vi "Reset Encoder_1.vi"(2 "DC Motors":cluster{"DC Motor":T1, "Address":i16}={"DC Motor"=enum."DC Motor", "Address"=-1}, 3 "NXT":T2={"Hardware"="NXT", "Flattened String"=""}) -> (0 "NXT":T2={"Hardware"="NXT", "Flattened String"=""})   [LabVIEW 2010, in "4134Outputs.lvlib"]
uses:
  4134Outputs.lvlib
  <vilib>/NXT/Subs/LVHSConnector.ctl
  <vilib>/NXT/Subs/MotorXNode.DC Motor Type.ctl
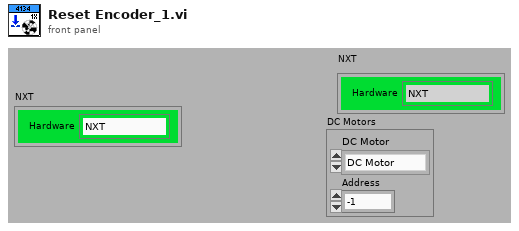
[diagram p1: front panel]
types:
  T1 = typedef "MotorXNode.DC Motor Type.ctl" = enum16{"DC Motor"}
  T2 = typedef "LVHSConnector.ctl" = cluster{"Hardware":string, "Flattened String":string}
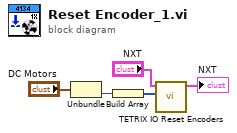
[diagram p0: block diagram]
diagram:
  n1 = Unbundle("DC Motors") -> ("Address"=w5:i16)  [unwired: 1 out]
  n2 = Build Array(w5) -> (w2:i16[])
  n3 = call <vilib>:"TETRIX IO Reset Encoders.vi"("DC Motors"=w2, "NXT"="NXT") -> ("NXT"=→"NXT":T2)  [unwired: 9 in]
